vi "RECIPE_NAME_UPLOAD.vi"(0 "CtlRef":refnum<vi>, 1 "Cluster":T1={"IP Address"=["", "", "", "", "", "", "", "", "", ""], "Machine name"=["", "", "", "", "", "", "", "", "", ""], "Station number"=["", "", "", "", "", "", "", "", "", ""], "Product List"=[], "Recipe_upload_history path"=path "", "reference"=refnum, "appended array"=[]}, 3 "error in (no error)":errorcluster) -> (7 "Recipe Names INDEX":i32[](array[numeric]), 8 "Recipe Names":string[](array[string]), 10 "error out":errorcluster)   [LabVIEW 2017]
uses:
  Controls/cluster.ctl
  <vilib>/addons/database/Connection.llb/Conn ObjectReference.ctl
  <vilib>/addons/database/NI_Database_API.lvlib
panel:
  in  "PRODUCT LIST":string(combo)
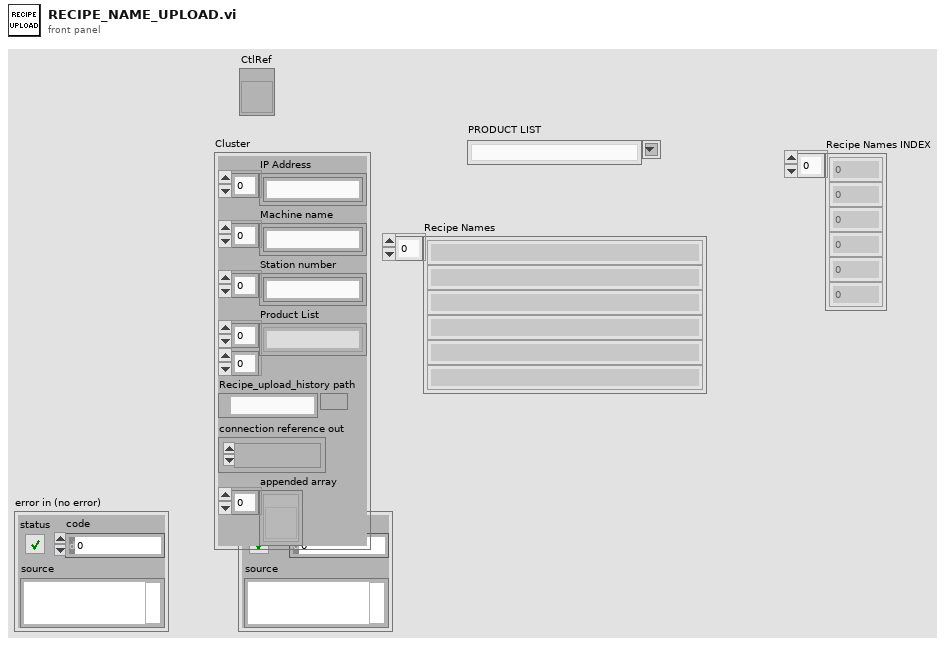
[diagram p1: front panel]
types:
  T1 = typedef "cluster.ctl" = cluster{"IP Address":string[], "Machine name":string[], "Station number":string[], "Product List":string[][], "Recipe_upload_history path":path, "reference":T2, "appended array":refnum<vi>[]}
  T2 = typedef "NI_Database_API.lvlib/Conn ObjectReference.ctl" = refnum<k1>
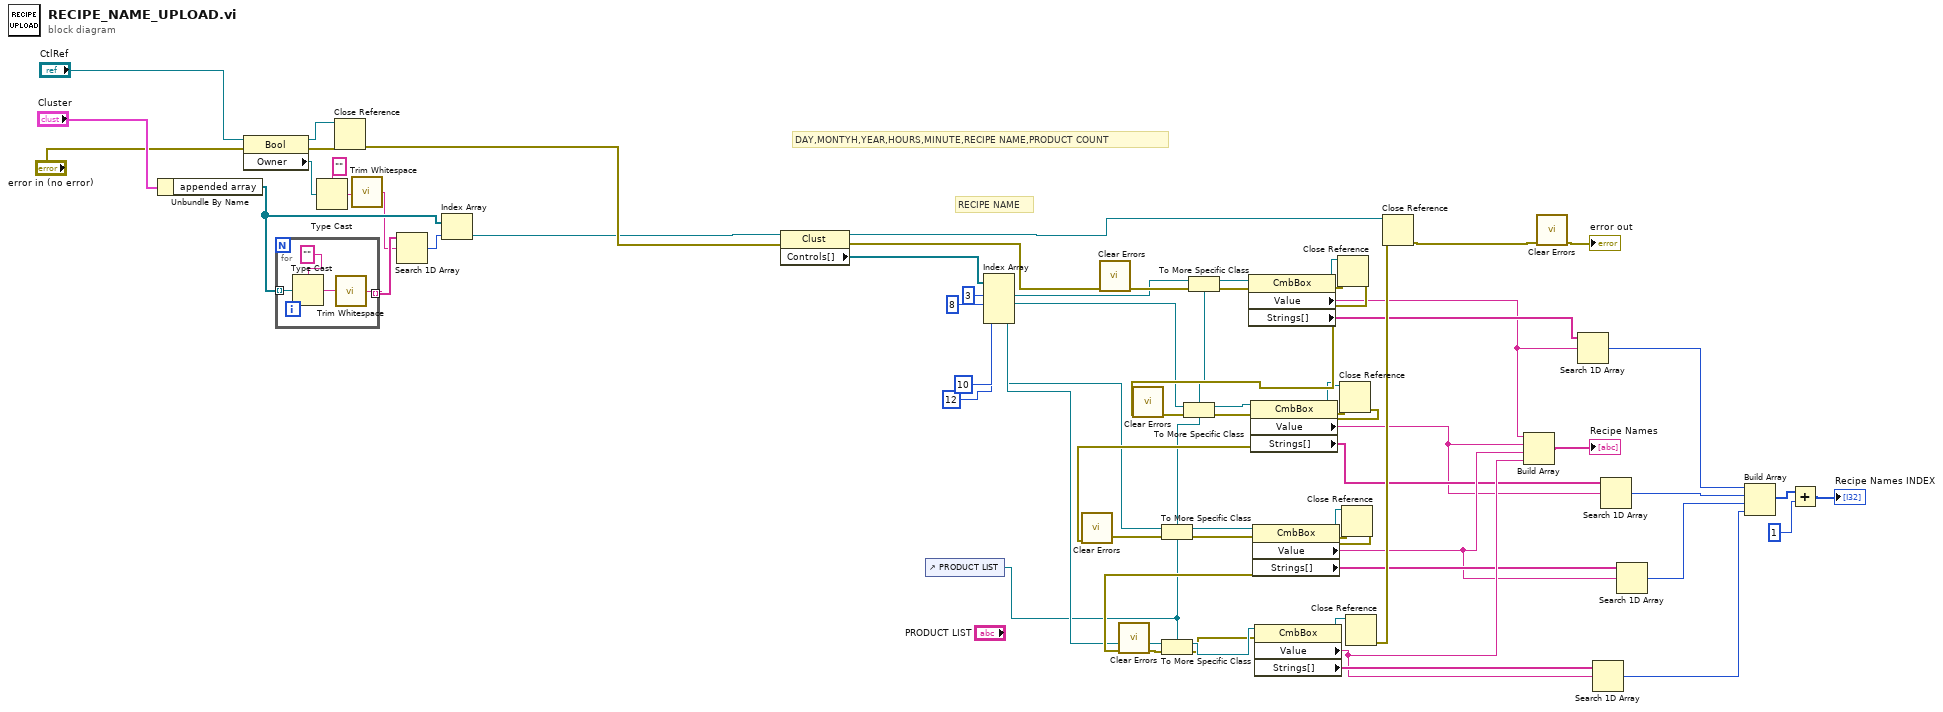
[diagram p0: block diagram]
diagram:
  # "RECIPE NAME"
  # "DAY,MONTYH,YEAR,HOURS,MINUTE,RECIPE NAME,PRODUCT COUNT"
  n1 = Unbundle By Name("Cluster") -> ("appended array"=w67:refnum<vi>[])
  n2 = property class="Bool"(reference="CtlRef", error in="error in (no error)") -> (reference out=w59:refnum<vi>, error out=w60:errorcluster, "Owner"=w63:refnum<vi>)
  n3 = for {
    tunnel: w67 -> [w71] mode=indexing
    tunnel: [w68] -> w65 mode=indexing
    n4 = Type Cast(type="" ("String"), x=w71) -> (*(type *) &x=w69:string)
    n5 = call <vilib>:"Trim Whitespace.vi"("string"=w69) -> ("trimmed string"=w68:string)  [unwired: 1 in]
  }
  n6 = Type Cast(type="", x=w63) -> (*(type *) &x=w62:string)
  n7 = Close Reference(reference=w59, error in (no error)=w60) -> (error out=w56:errorcluster)
  n8 = call <vilib>:"Trim Whitespace.vi"("string"=w62) -> ("trimmed string"=w64:string)  [unwired: 1 in]
  n9 = Search 1D Array(1D array=w65, element=w64) -> (index of element=w66:i32)  [unwired: 1 in]
  n10 = Index Array(array=w67, index=w66) -> (element=w54:refnum<vi>)
  n11 = property class="Clust"(reference=w54, error in=w56) -> (reference out=w52:refnum<vi>, error out=w53:errorcluster, "Controls[]"=w50:refnum<vi>[])
  n12 = control-ref of="PRODUCT LIST"() -> (w19:refnum<vi>)
  n13 = Index Array(array=w50, index #1=3 ("index"), index #2=8 ("index"), index #3=10 ("index"), index #4=12 ("index")) -> (element #1=w20:refnum<vi>, element #2=w24:refnum<vi>, element #3=w29:refnum<vi>, element #4=w36:refnum<vi>)
  n14 = call <vilib>:"Clear Errors.vi"("error in (no error)"=w53) -> ("error out"=w23:errorcluster)  [unwired: 5 in, 1 out]
  n15 = To More Specific Class(target class=w19, reference=w20, error in=w23) -> (specific class reference=w21:refnum<vi>, error out=w22:errorcluster)
  n16 = property class="CmbBox"(reference=w21, error in=w22) -> (reference out=w39:refnum<vi>, error out=w51:errorcluster, "Value"=w8:string, "Strings[]"=w9:string[])
  n17 = Close Reference(reference=w39, error in (no error)=w51) -> (error out=w42:errorcluster)
  n18 = call <vilib>:"Clear Errors.vi"("error in (no error)"=w42) -> ("error out"=w27:errorcluster)  [unwired: 5 in, 1 out]
  n19 = To More Specific Class(target class=w19, reference=w24, error in=w27) -> (specific class reference=w25:refnum<vi>, error out=w26:errorcluster)
  n20 = property class="CmbBox"(reference=w25, error in=w26) -> (reference out=w38:refnum<vi>, error out=w45:errorcluster, "Value"=w10:string, "Strings[]"=w11:string[])
  n21 = Close Reference(reference=w38, error in (no error)=w45) -> (error out=w41:errorcluster)
  n22 = call <vilib>:"Clear Errors.vi"("error in (no error)"=w41) -> ("error out"=w30:errorcluster)  [unwired: 5 in, 1 out]
  n23 = To More Specific Class(target class=w19, reference=w29, error in=w30) -> (specific class reference=w28:refnum<vi>, error out=w31:errorcluster)
  n24 = property class="CmbBox"(reference=w28, error in=w31) -> (reference out=w37:refnum<vi>, error out=w44:errorcluster, "Value"=w12:string, "Strings[]"=w13:string[])
  n25 = Close Reference(reference=w37, error in (no error)=w44) -> (error out=w40:errorcluster)
  n26 = call <vilib>:"Clear Errors.vi"("error in (no error)"=w40) -> ("error out"=w33:errorcluster)  [unwired: 5 in, 1 out]
  n27 = To More Specific Class(target class=w19, reference=w36, error in=w33) -> (specific class reference=w34:refnum<vi>, error out=w32:errorcluster)
  n28 = property on="Property Node" class="CmbBox"(reference=w34, error in=w32) -> (reference out=w35:refnum<vi>, "Value"=w14:string, "Strings[]"=w15:string[])  [unwired: 1 out]
  n29 = Close Reference(reference=w35) -> (error out=w43:errorcluster)  [unwired: 1 in]
  n30 = Close Reference(reference=w52, error in (no error)=w43) -> (error out=w17:errorcluster)
  n31 = Build Array(w8, w10, w12, w14) -> (→"Recipe Names":string[])
  n32 = call <vilib>:"Clear Errors.vi"("error in (no error)"=w17) -> ("error out"=→"error out":errorcluster)  [unwired: 5 in, 1 out]
  n33 = Search 1D Array(1D array=w9, element=w8) -> (index of element=w7:i32)  [unwired: 1 in]
  n34 = Search 1D Array(1D array=w15, element=w14) -> (index of element=w4:i32)  [unwired: 1 in]
  n35 = Search 1D Array(1D array=w11, element=w10) -> (index of element=w6:i32)  [unwired: 1 in]
  n36 = Search 1D Array(1D array=w13, element=w12) -> (index of element=w5:i32)  [unwired: 1 in]
  n37 = Build Array(w7, w6, w5, w4) -> (w3:i32[])
  n38 = Add(x=w3, y=1 ("index of element")) -> (x+y=→"Recipe Names INDEX":i32[])
